vi "network stream write.vi"(8 "error in (no error)":errorcluster, 10 "Data":fxp<+/-,17,5> format="%#_17g", 11 "endpoint in":refnum<k21>) -> (0 "error out":errorcluster, 3 "endpoint out":refnum<k21>)   [LabVIEW 2017]
uses:
  <resource>/objmgr/ni.dex.rc
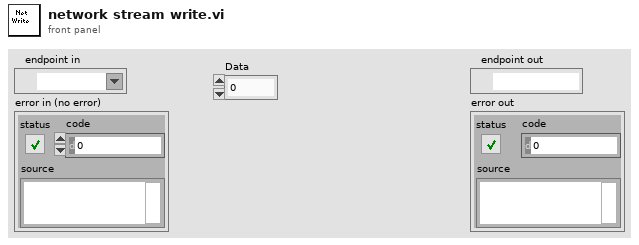
[diagram p1: front panel]
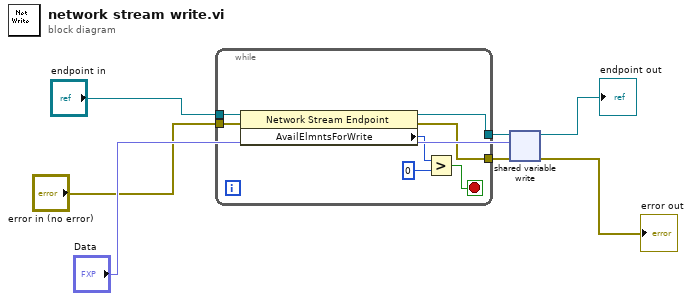
[diagram p0: block diagram]
diagram:
  n1 = while {
    tunnel: "endpoint in" -> [w14]
    tunnel: "error in (no error)" -> [w13]
    tunnel: [w9] -> w4
    tunnel: [w8] -> w3
    stop <- w10 stop-if-true
    n2 = property class="Network Stream Endpoint"(reference=w14, error in=w13) -> (reference out=w9:refnum<k21>, error out=w8:errorcluster, "AvailElmntsForWrite"=w12:i32)
    n3 = Greater?(x=w12, y=0) -> (0:w10:bool)
  }
  n4 = shared-variable-write(w4, w3, "Data") -> (→"endpoint out":refnum<k21>, →"error out":errorcluster)  [unwired: 1 in, 1 out]
